vi "LaserOnOff.vi"(10 "Laser on/off":bool, 11 "client handle in":T1) -> (2 "LaserOn?":bool, 3 "client handle out":T1)   [LabVIEW 2020]
uses:
  <vilib>/httpClient/ClientHandle.ctl
  <vilib>/JDP Science/JSONtext/String Subset.vi
  <vilib>/JDP Science/JSONtext/Parsing/Parse Full Path or Item Name.vi
  <vilib>/JDP Science/JSONtext/Next JSON Value.vi
  <vilib>/JDP Science/JSONtext/support/Error Cluster From Code.vi
  <vilib>/JDP Science/JSONtext/Offset/Find Item Locations by Path.vi
  <vilib>/httpClient/LabVIEWHTTPClient.lvlib
  <vilib>/wsapi/NI_WebServices.lvlib
  <vilib>/JDP Science/JSONtext/JSONtext.lvlib
panel:
  out "body":string
  out "headers":string
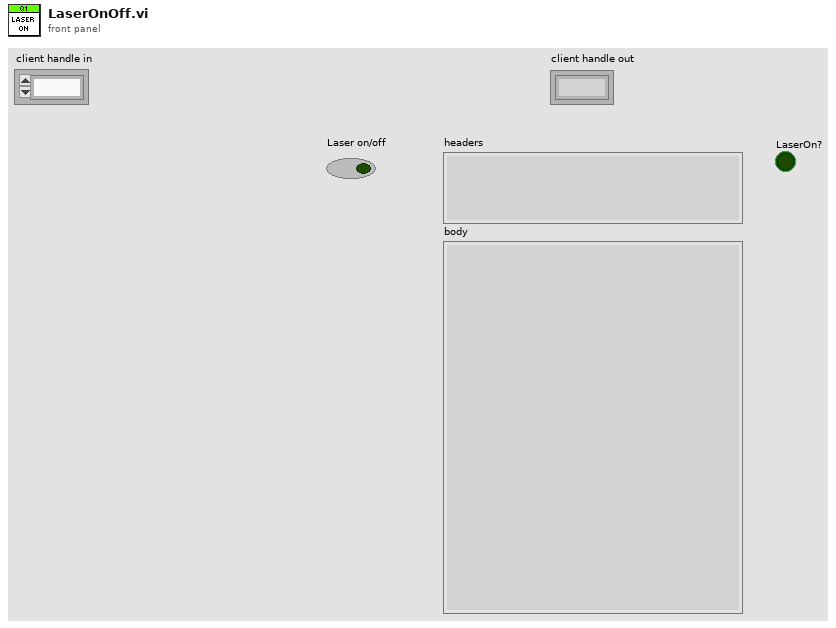
[diagram p1: front panel]
types:
  T1 = typedef "LabVIEWHTTPClient.lvlib/ClientHandle.ctl" = refnum<k1>
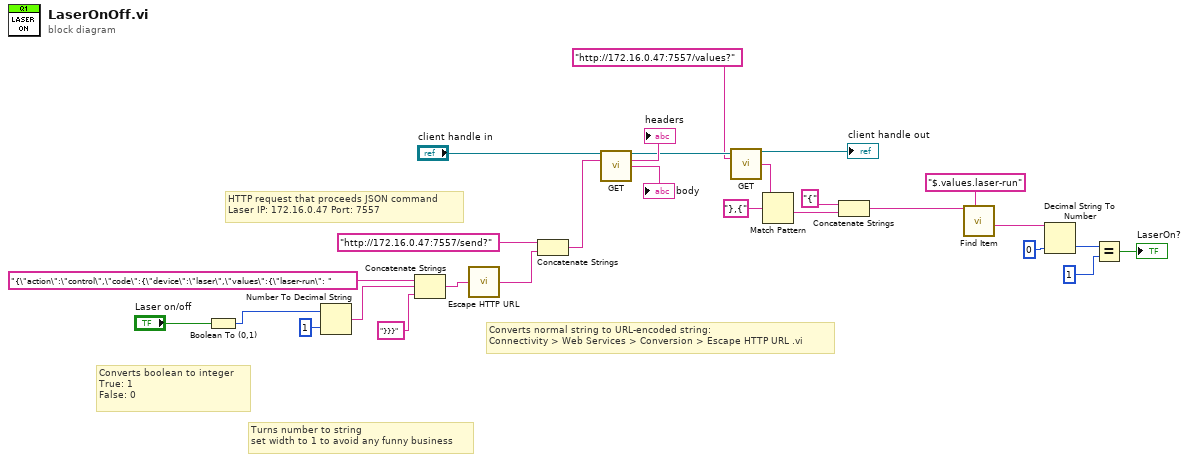
[diagram p0: block diagram]
diagram:
  # "Turns number to string\nset width to 1 to avoid any funny business"
  # "Converts boolean to integer \nTrue: 1\nFalse: 0"
  # "Converts normal string to URL-encoded string:\nConnectivity > Web Services > Conversion > Escape HTTP URL .vi"
  # "HTTP request that proceeds JSON command\nLaser IP: 172.16.0.47 Port: 7557"
  n1 = Boolean To (0,1)(Boolean="Laser on/off") -> (0, 1=w4:i16)
  n2 = Number To Decimal String(number=w4, width (-)=i16 1) -> (decimal integer string=w6:string)
  n3 = Concatenate Strings("{\"action\":\"control\",\"code\":{\"device\":\"laser\",\"values\":{\"laser-run\": " ("JSON command"), w6, "}}}" ("string")) -> (w9:string)
  n4 = call <vilib>:"Escape HTTP URL.vi"("unescaped string in"=w9) -> ("escaped string out"=w23:string)
  n5 = Concatenate Strings("http://172.16.0.47:7557/send?", w23) -> (w25:string)
  n6 = call <vilib>:"GET.vi"("client handle"="client handle in", "url"=w25) -> ("client handle out"=w18:T1, "headers"=→"headers":string, "body"=→"body":string)  [unwired: 10 in, 1 out]
  n7 = call <vilib>:"GET.vi"("client handle"=w18, "url"="http://172.16.0.47:7557/values?") -> ("client handle out"=→"client handle out":T1, "body"=w19:string)  [unwired: 10 in, 2 out]
  n8 = Match Pattern(string=w19, regular expression="},{") -> (after substring=w20:string)  [unwired: 1 in, 3 out]
  n9 = Concatenate Strings("{" ("string"), w20) -> (w12:string)
  n10 = call <vilib>:"Find Item.vi"("$Path or Item Name"="$.values.laser-run", "JSON"=w12) -> ("<JSON>"=w15:string)  [unwired: 6 in, 3 out]
  n11 = Decimal String To Number(string=w15, default (0L)=0 ("default (0 I32)")) -> (number=w13:i32)  [unwired: 1 in, 1 out]
  n12 = Equal?(x=w13, y=1) -> (x = y?=→"LaserOn?":bool)
